vi "mergetest.vi"(10 "Array of Points":T1[](array[typedef])=[{"X Pos"=30.0, "Y Pos"=10.0, "Bearing"=0.0}, {"X Pos"=40.0, "Y Pos"=20.0, "Bearing"=0.0}, {"X Pos"=30.0, "Y Pos"=30.0, "Bearing"=0.0}, {"X Pos"=30.0, "Y Pos"=40.0, "Bearing"=0.0}, {"X Pos"=40.0, "Y Pos"=50.0, "Bearing"=0.0}, {"X Pos"=40.0, "Y Pos"=60.0, "Bearing"=0.0}, {"X Pos"=30.0, "Y Pos"=60.0, "Bearing"=0.0}]) -> ()   [LabVIEW 2017]
uses:
  040-typeDefs/Position.ctl
  <vilib>/addons/control/pid/pid.llb/PID (DBL).vi
  <vilib>/addons/control/pid/NI_PID_pid.lvlib
panel:
  in  "stop":bool
  out "XY Graph 2":cluster{"X":dbl, "Y":dbl}[](graph)
  out "Array":bool[](array[boolean])
  out "Distance from destination":dbl(graph)=8.541298456610324
  out "X, Y, BEARING":cluster{dbl, dbl, dbl}
  out "radius":dbl=-740.4944109617504
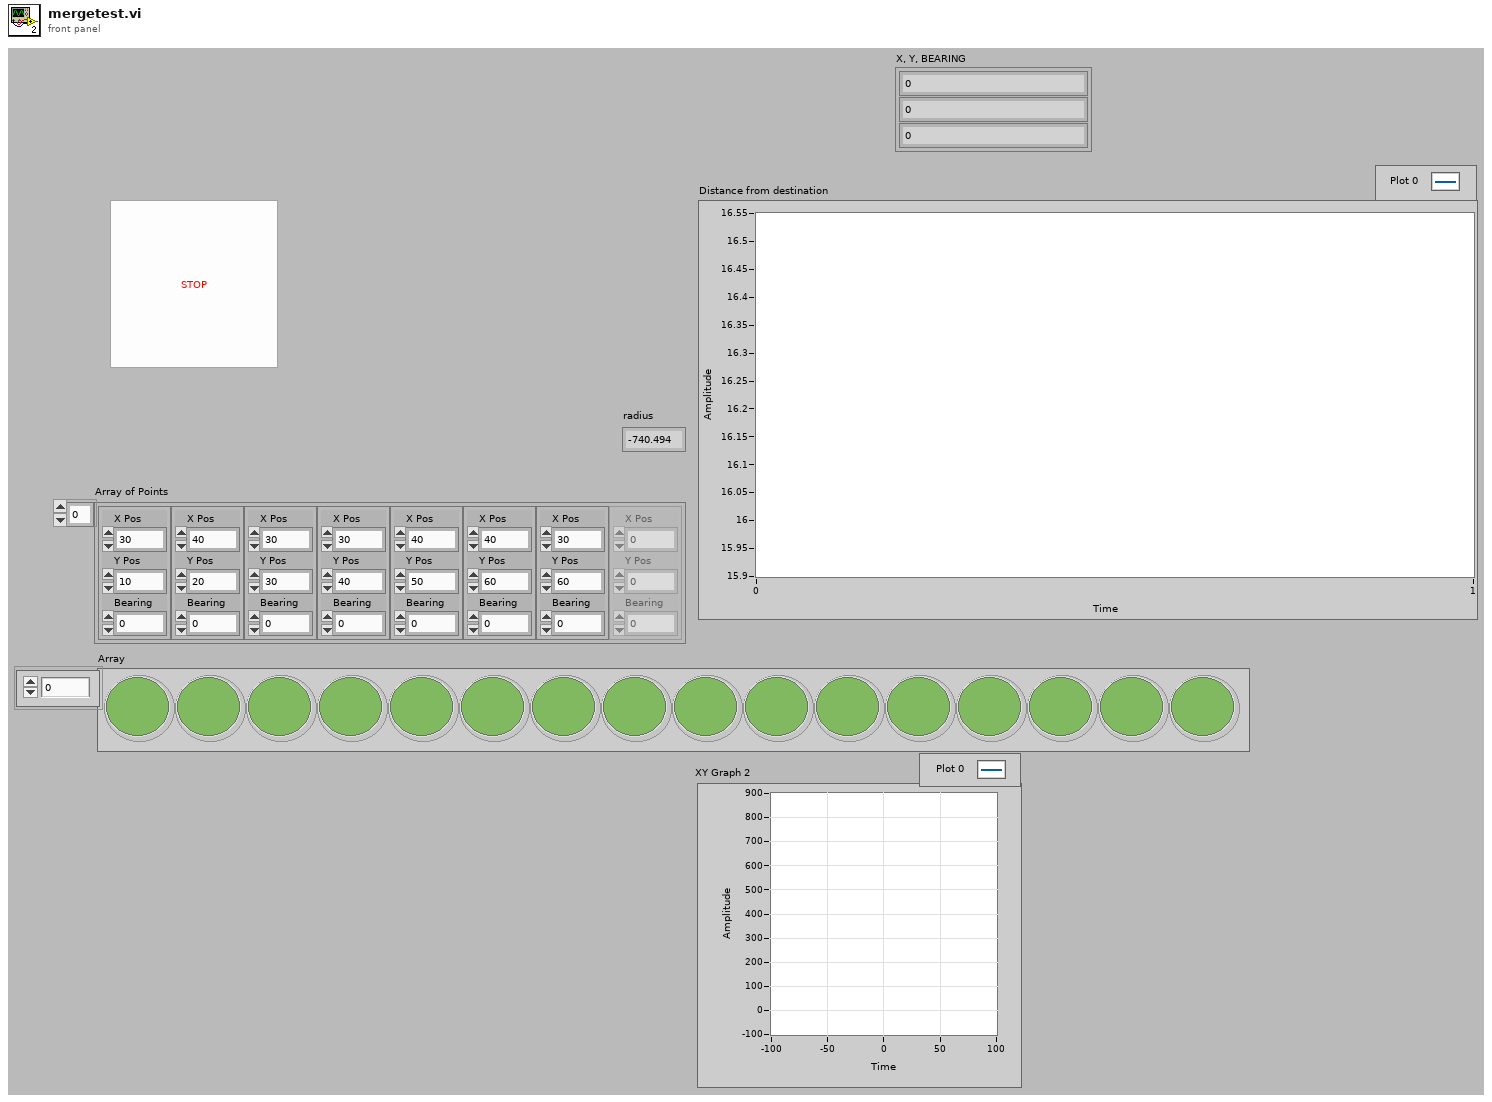
[diagram p1: front panel]
types:
  T1 = typedef "Position.ctl" = cluster{"X Pos":dbl, "Y Pos":dbl, "Bearing":dbl}
  T2 = cluster{"proportional gain (Kc)":dbl, "integral time (Ti, min)":dbl, "derivative time (Td, min)":dbl}
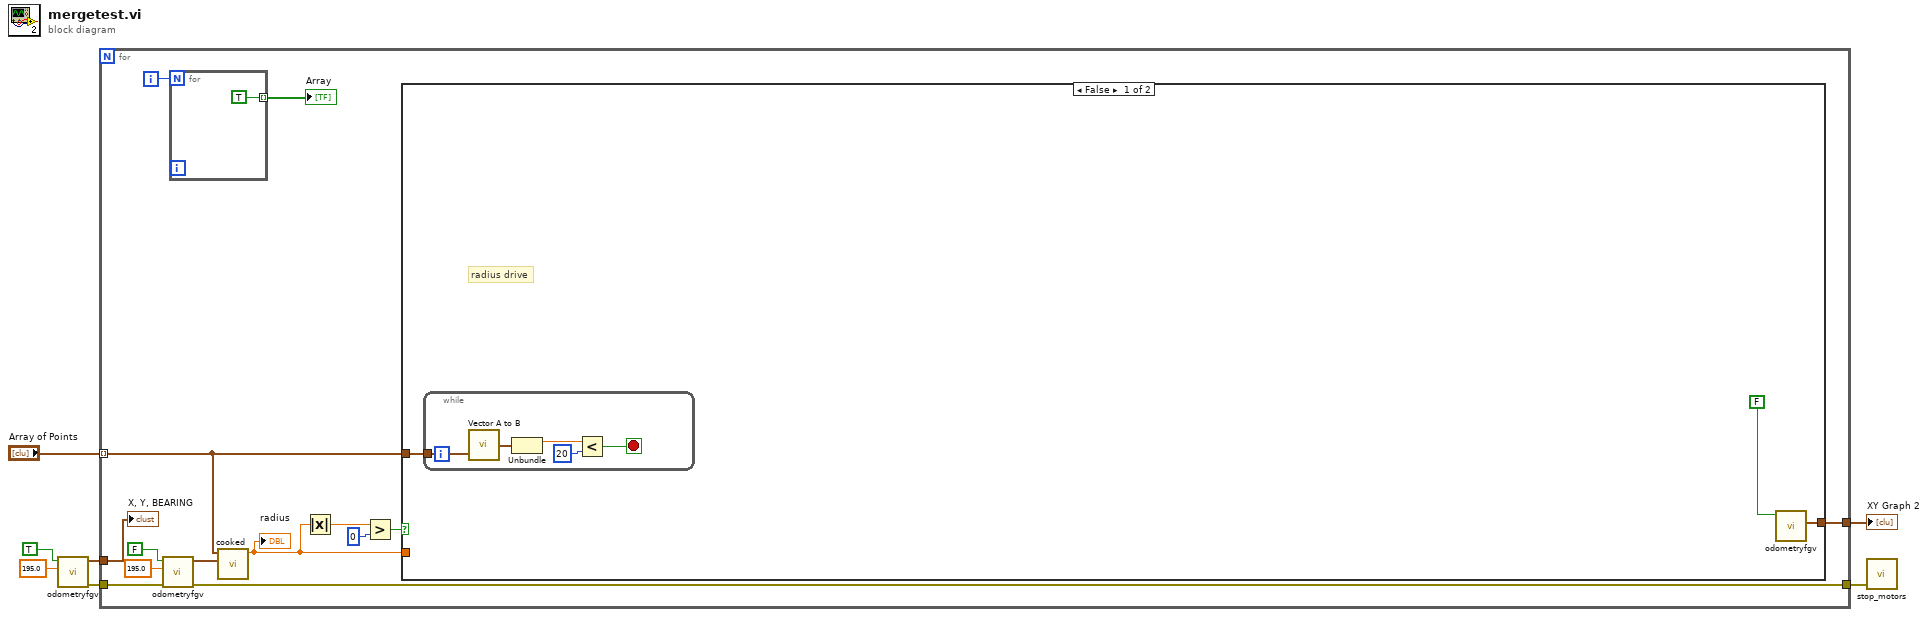
[diagram p0: block diagram]
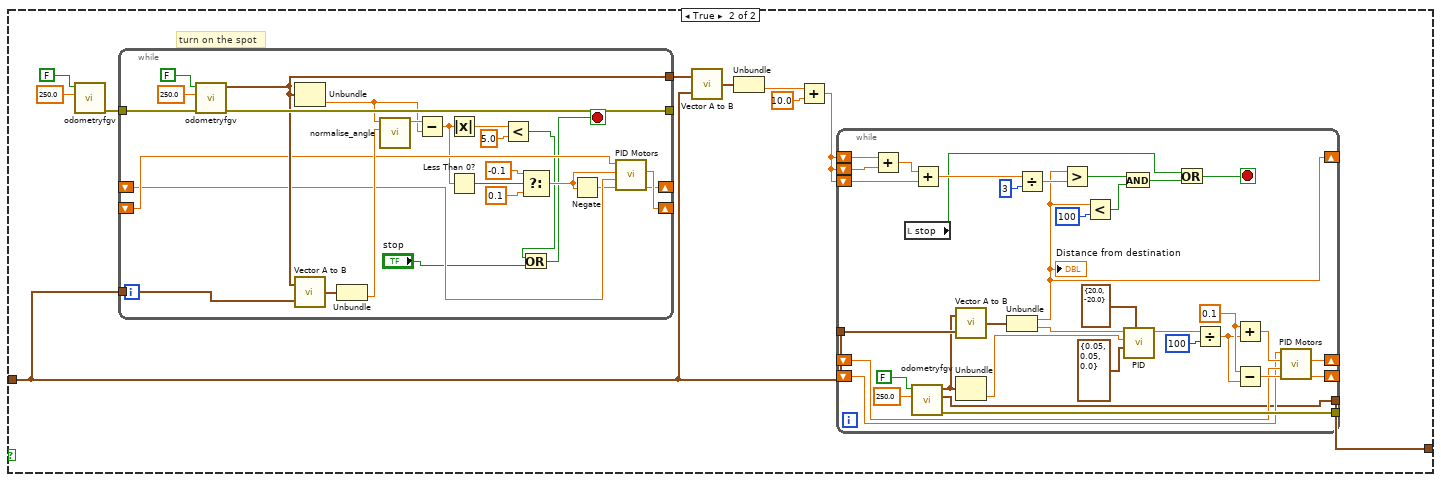
[diagram p2: hidden frame]
diagram:
  n1 = call "odometryfgv.vi"("wheelbase"=195.0, "Reset"=TRUE) -> ("error out"=w4:errorcluster, "X, Y, BEARING"=w3:cluster{dbl, dbl, dbl})  [unwired: 6 in, 1 out]
  n2 = for {
    tunnel: "Array of Points" -> [w21] mode=indexing
    tunnel: w4 -> [w20]
    tunnel: w3 -> [w19]
    tunnel: [w18] -> w2
    tunnel: [w8] -> w1
    i -> [w17]
    n3 = call "odometryfgv.vi"("error in (no error)"=w20, "wheelbase"=195.0, "Reset"=FALSE) -> ("error out"=w18:errorcluster, "X, Y, BEARING"=w10:cluster{dbl, dbl, dbl})  [unwired: 5 in, 1 out]
    n4 = for {
      N: w17 -> [_]
      tunnel: [TRUE] -> w16 mode=indexing
    }
    "Array" <- w16
    n5 = call "cooked.vi"("destination"=w10, "current"=w21) -> ("Numeric"=w9:dbl)  [unwired: 9 in]
    "radius" <- w9
    n6 = Absolute Value(x=w9) -> (abs(x)=w11:dbl)
    n7 = Greater?(x=w11, y=0) -> (0:w12:bool)
    n8 = case shown="False" w12 {
      tunnel: w21 -> [w24 w33]
      tunnel: w9 -> [_ _]
      tunnel: [w23 w39] -> w8
      frame False {
        # "radius drive"
        n9 = while {
          tunnel: w24 -> [w28]
          stop <- w25 stop-if-true
          n10 = call "Vector A to B.vi"("Destination"=w28) -> ("vector"=w29:cluster{dbl, "Bearing":dbl})  [unwired: 1 in]
          n11 = Unbundle(w29) -> (w27:dbl)  [unwired: 1 out]
          n12 = Less?(x=w27, y=20) -> (x < y?=w25:bool)
        }
        n13 = call "odometryfgv.vi"("Reset"=FALSE) -> ("XY Graph 2"=w23:cluster{"X":dbl, "Y":dbl}[])  [unwired: 7 in, 2 out]
      }
      frame True {
        # "turn on the spot"
        n14 = call "odometryfgv.vi"("wheelbase"=250.0, "Reset"=FALSE) -> ("error out"=w34:errorcluster)  [unwired: 6 in, 2 out]
        n15 = while {
          tunnel: w33 -> [w95]
          tunnel: w34 -> [w97]
          tunnel: [w96] -> _
          tunnel: [w92] -> w31
          shift-right: [w88] -> _
          shift-left: _ -> [w86]
          shift-right: [w89] -> _
          shift-left: _ -> [w87]
          stop <- w76 stop-if-true
          n16 = call "odometryfgv.vi"("error in (no error)"=w97, "wheelbase"=250.0, "Reset"=FALSE) -> ("error out"=w96:errorcluster, "X, Y, BEARING"=w92:cluster{dbl, dbl, dbl})  [unwired: 5 in, 1 out]
          n17 = Unbundle(w92) -> (w90:dbl)  [unwired: 2 out]
          n18 = call "Vector A to B.vi"("Destination"=w95, "Current"=w92) -> ("vector"=w94:cluster{dbl, "Bearing":dbl})
          n19 = Unbundle(w94) -> ("Bearing"=w93:dbl)  [unwired: 1 out]
          n20 = call "normalise_angle.vi"("target -180 .. 180"=w93, "current"=w90) -> ("travel_direction"=w91:dbl)  [unwired: 9 in]
          n21 = Subtract(x=w91, y=w90) -> (x-y=w80:dbl)
          n22 = Absolute Value(x=w80) -> (abs(x)=w79:dbl)
          n23 = Less Than 0?(x=w80) -> (x < 0?=w84:bool)
          n24 = Less?(x=w79, y=5.0) -> (x < y?=w77:bool)
          n25 = Select(t=-0.1, s=w84, f=0.1) -> (s? t:f=w81:dbl)
          n26 = Or(x=w77, y="stop") -> (x .or. y?=w76:bool)
          n27 = Negate(x=w81) -> (-x=w85:dbl)
          n28 = call "PID Motors.vi"("input B"=w85, "Speed B"=w86, "input A"=w81, "Speed A"=w87) -> ("output B"=w88:dbl, "output A"=w89:dbl)  [unwired: 2 out]
        }
        n29 = call "Vector A to B.vi"("Destination"=w33, "Current"=w31) -> ("vector"=w32:cluster{dbl, "Bearing":dbl})
        n30 = Unbundle(w32) -> ("Bearing"=w30:dbl)  [unwired: 1 out]
        n31 = Add(x=w30, y=10.0) -> (x+y=w36:dbl)
        n32 = while {
          tunnel: w33 -> [w74]
          shift-right: [w71] -> _
          shift-left: _ -> [w61]
          shift-right: [w72] -> _
          shift-left: _ -> [w62]
          tunnel: [w65] -> _
          tunnel: [w55] -> w39
          shift-right: [w42] -> _
          shift-left: w36 -> [w54]
          shift-left: w36 -> [w53]
          shift-left: w36 -> [w51]
          stop <- w60 stop-if-true
          w66 = 0.1
          n33 = Add(x=w54, y=w53) -> (x+y=w52:dbl)
          n34 = local read "stop"() -> (w40:bool)
          n35 = call "odometryfgv.vi"("wheelbase"=250.0, "Reset"=FALSE) -> ("error out"=w65:errorcluster, "XY Graph 2"=w55:cluster{"X":dbl, "Y":dbl}[], "X, Y, BEARING"=w69:cluster{dbl, dbl, dbl})  [unwired: 6 in]
          n36 = Add(x=w52, y=w51) -> (x+y=w50:dbl)
          n37 = call "Vector A to B.vi"("Destination"=w74, "Current"=w69) -> ("vector"=w73:cluster{dbl, "Bearing":dbl})
          n38 = Unbundle(w69) -> (w68:dbl)  [unwired: 2 out]
          n39 = Unbundle(w73) -> (w42:dbl, "Bearing"=w70:dbl)
          "Distance from destination" <- w42
          n40 = Divide(x=w50, y=3) -> (x/y=w46:dbl)
          n41 = Greater?(x=w42, y=w46) -> (0:w45:bool)
          n42 = Less?(x=w42, y=100) -> (x < y?=w43:bool)
          n43 = And(x=w45, y=w43) -> (x .and. y?=w44:bool)
          n44 = call-poly <vilib>:"PID.vi"("output range"=cluster{"output high":dbl, "output low":dbl} {"output high"=20.0, "output low"=-20.0}, "PID gains"=T2 {"proportional gain (Kc)"=0.05, "integral time (Ti, min)"=0.05, "derivative time (Td, min)"=0.0}, "process variable"=w68, "setpoint"=w70) -> ("output"=w58:dbl)  [unwired: 6 in, 1 out]
          n45 = Or(x=w40, y=w44) -> (x .or. y?=w60:bool)
          n46 = Divide(x=w58, y=100) -> (x/y=w56:dbl)
          n47 = Add(x=w66, y=w56) -> (x+y=w64:dbl)
          n48 = Subtract(x=w66, y=w56) -> (x-y=w63:dbl)
          n49 = call "PID Motors.vi"("input B"=w63, "Speed B"=w62, "input A"=w64, "Speed A"=w61) -> ("output B"=w71:dbl, "output A"=w72:dbl)  [unwired: 2 out]
        }
      }
    }
    "X, Y, BEARING" <- w19
  }
  "XY Graph 2" <- w1
  n50 = call "stop_motors.vi"("error in (no error)"=w2) -> ()  [unwired: 4 in, 1 out]
